vi "AuMT8852B Initial Carrier Test Configuration.vi"(5 "Settings":T1={"Low frequency selection"=enum."Use low frequency", "Medium frequency selection"=enum."Use medium frequency", "High frequency selection"=enum."Use high frequency", "Low TX frequency"=2402.0, "Medium TX frequency"=2441.0, "High TX frequency"=2480.0, "Number of packets"=10, "Hop selection"=enum."Test with hopping on", "Hop mode"=enum."Defined", "Test control"=enum."Loopback", "Maximum positive limit"=75000.0, "Maximum negative limit"=75000.0, "Low RX frequency"=2480.0, "Medium RX frequency"=2402.0, "High RX frequency"=2402.0}, 7 "Set/Get (Set)":enum16{"Set", "Get"}(ring), 8 "error in (no error)":errorcluster, 10 "Script (3)":i32=3, 11 "VISA session":refnum<visa-resource-name>) -> (0 "error out":errorcluster, 2 "error code":i32, 3 "VISA session out":refnum<visa-resource-name>, 4 "Settings out":T1={"Low frequency selection"=enum."Use low frequency", "Medium frequency selection"=enum."Use medium frequency", "High frequency selection"=enum."Use high frequency", "Low TX frequency"=0.0, "Medium TX frequency"=0.0, "High TX frequency"=0.0, "Number of packets"=0, "Hop selection"=enum."Test with hopping on", "Hop mode"=enum."Any", "Test control"=enum."Loopback", "Maximum positive limit"=0.0, "Maximum negative limit"=0.0, "Low RX frequency"=0.0, "Medium RX frequency"=0.0, "High RX frequency"=0.0})   [LabVIEW 2017]
doc: "Anritsu MT8852B Bluetooth Tester\n\nConfigures the instrument for the Initial Carrier test.\n\nINPUTS\nSet/Get - whether the values are being sent to or retrieved from the instrument.\nScript - which of the stored scripts (1-10) will be queried or configured. Scripts 1 and 2 are read-only.\nSettings - parameters of the test to be written.\n\nOUTPUTS\nSettings out - current parameters of the test."
uses:
  <instrlib>/aumt8852B/General/Utilities/MT8850 Test Parameters.ctl
  <instrlib>/aumt8852B/General/Utilities/MT8850 Frequency Units.ctl
panel:
  in  "Case Constant\n(See Context Help)":bool
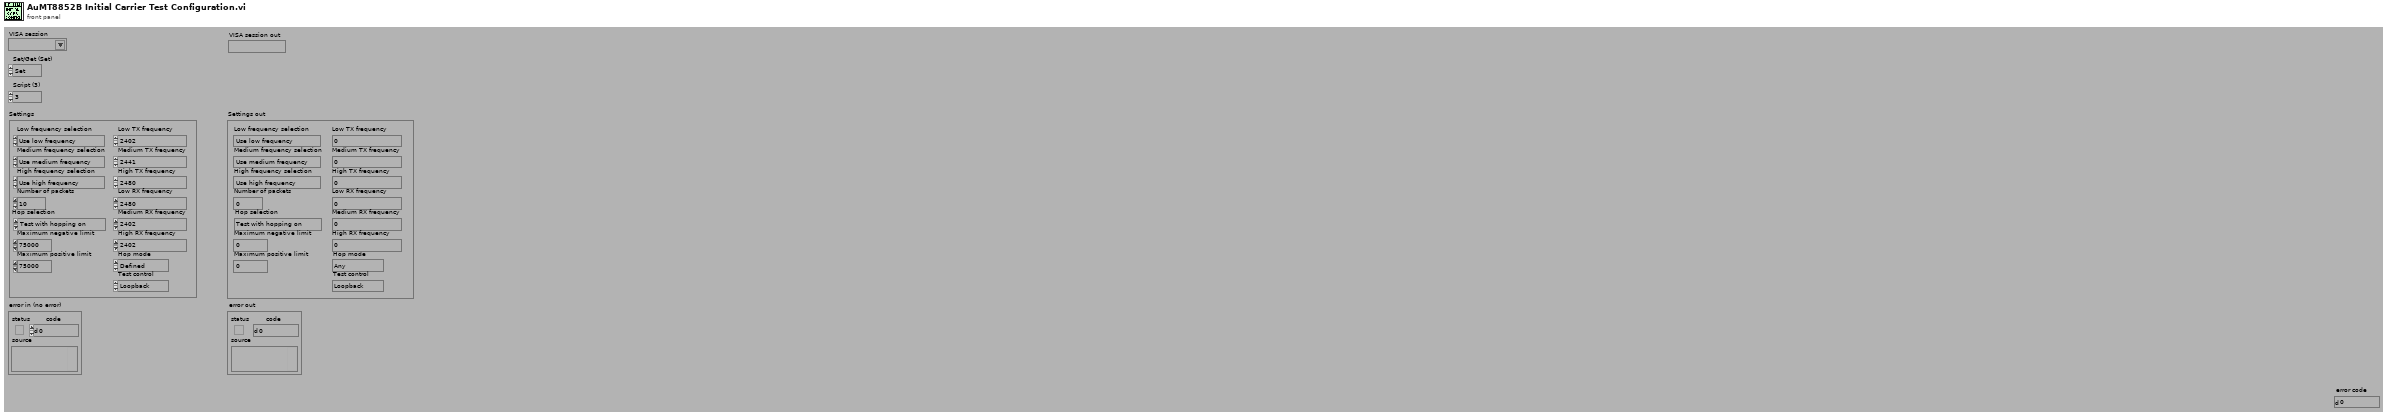
[diagram p1: front panel]
types:
  T1 = cluster{"Low frequency selection":enum16{"Don't use low frequency", "Use low frequency"}, "Medium frequency selection":enum16{"Don't use medium frequency", "Use medium frequency"}, "High frequency selection":enum16{"Don't use high frequency", "Use high frequency"}, "Low TX frequency":dbl, "Medium TX frequency":dbl, "High TX frequency":dbl, "Number of packets":i32, "Hop selection":enum16{"Test with hopping on", "Test with hopping off", "Test with hopping on and off"}, "Hop mode":enum16{"All", "Any", "Defined"}, "Test control":enum16{"Loopback", "TX test"}, "Maximum positive limit":dbl, "Maximum negative limit":dbl, "Low RX frequency":dbl, "Medium RX frequency":dbl, "High RX frequency":dbl}
  T2 = typedef "MT8850 Test Parameters.ctl" = enum16{"Use low frequency", "Use medium frequency", "Use high frequency", "Low TX frequency", "Low RX frquency", "Medium TX frequency", "Medium RX frequency", "High TX frequency", "High RX frequency", "Number of packets", "Average high limit", "Average low limit", "Peak power limit", "Max power step limit", "Min power step limit", "f1 average minimum", "f1 average maximum", "f2 maximum", "f1/f2 average maximum", "Hop selection", "Use DH1 packets", "Use DH3 packets", "Use DH5 packets", "1 slot packet drift limit", "3 slot packet drift limit", "5 slot packet drift limit", "Drift rate limit", "TX power level", "Frequency offset", "Symbol timing", "Modulation index", "BER limit", "FER limit", "Use averaging high limit", "Use averaging low limit", "Use peak power limit", "Packet type", "Test control", "Use max power step limit", "Use min power step limit", "Number of cycles", "Use f1 average maximum", "Use f1 average minimum", "Use f2 maximum", "Use f1/f2 average maximum", "Hop mode", "Maximum negative limit", "Maximum positive limit", "Use maximum negative limit", "Use maximum positive limit", "Use 1 slot packet drift limit", "Use 3 slot packet drift limit", "Use 5 slot packet drift limit", "Use drift rate limit", "Use BER limit", "Use FER limit", "Use dirty parameter table", "Use null packet drift limit", "Null packet drift limit", "Minimum power", "Power delay", "Packet count", "Payload toggle", "Output power level", "2DHX packet type", "3DHX packet type", "Number of blocks", "TX and RX low frequency", "TX and RX medium frequency", "TX and RX high frequency", "TX frequency", "RX frequency", "Threshold bit count", "Total test bit count", "Number of bits", "PDPSK to PGFSK lower limit", "PDPSK to PGFSK upper limit", "Initial frequency error upper limit", "Initial frequency error lower limit", "Frequency error upper limit", "Frequency error lower limit", "Block frequency error upper limit", "Block frequency error lower limit", "2Mbs RMS DEVM limit", "3Mbs RMS DEVM limit", "2Mbs Peak DEVM limit", "3Mbs Peak DEVM limit", "2Mbs 99% packets DEVM limit", "3Mbs 99% packets DEVM limit", "Percentage of no error packets limit", "Threshold error limit", "Total test error limit"}
  T3 = typedef "MT8850 Frequency Units.ctl" = enum16{"Channel", "Hz", "kHz", "MHz", "GHz"}
  T4 = enum16{"Simulate", "Range check", "Cache", "Query instrument status"}
  T5 = enum16{"Output power", "Power control", "Modulation characteristics", "Initial carrier", "Carrier drift", "Single slot sensitivity", "Multiple slot sensitivity", "Maximum input power"}
  T6 = enum16{"Test with hopping on", "Test with hopping off", "Test with hopping on and off"}
  T7 = enum16{"Don't use high frequency", "Use high frequency"}
  T8 = enum16{"Don't use medium frequency", "Use medium frequency"}
  T9 = enum16{"Don't use low frequency", "Use low frequency"}
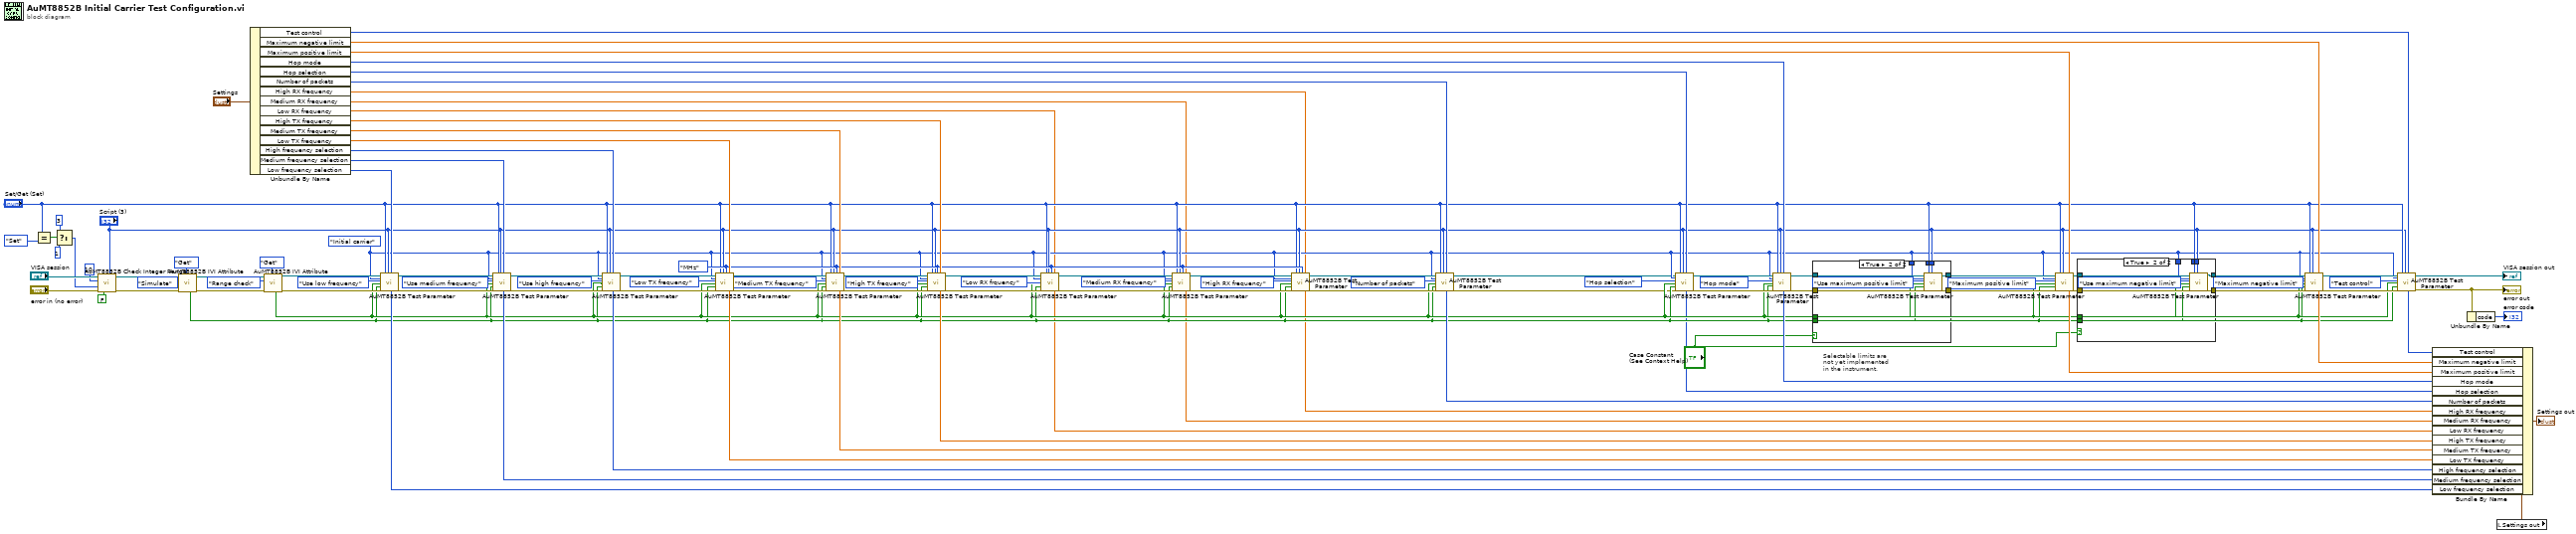
[diagram p0: block diagram]
diagram:
  w15 = MT8850_Frequency_Units."MHz" ("Frequency units (MHz)")
  w10 = T5."Initial carrier" ("Test (Output Power)")
  # "Selectable limits are\nnot yet implemented\nin the instrument."
  n1 = Equal?(x="Set/Get (Set)", y=enum16{"Set", "Get"}."Set") -> (x = y?=w106:bool)
  n2 = Select(t=3, s=w106, f=1) -> (s? t:f=w102:i32)
  n3 = call <instrlib>:"AuMT8852B Check Integer Range.vi"("Value (0)"="Script (3)", "Check IVI flag first? (T)"=FALSE, "error in (no error)"="error in (no error)", "Lower limit (-1)"=w102, "Upper limit (1)"=10, "VISA session"="VISA session") -> ("error out"=w100:errorcluster, "VISA session out"=w101:refnum<visa-resource-name>)  [unwired: 4 in]
  n4 = call <instrlib>:"AuMT8852B IVI Attribute.vi"("Set/Get (Set)"=enum16{"Set", "Get"}."Get", "error in (no error)"=w100, "Flag (Simulate)"=T4."Simulate", "VISA session"=w101) -> ("error out"=w81:errorcluster, "VISA session out"=w82:refnum<visa-resource-name>, "Value out"=w13:bool)  [unwired: 5 in]
  n5 = Unbundle By Name("Settings") -> ("Test control"=w43:enum16{"Loopback", "TX test"}, "Maximum negative limit"=w42:dbl, "Maximum positive limit"=w41:dbl, "Hop mode"=w60:enum16{"All", "Any", "Defined"}, "Hop selection"=w59:T6, "Number of packets"=w69:i32, "High RX frequency"=w9:dbl, "Medium RX frequency"=w8:dbl, "Low RX frequency"=w7:dbl, "High TX frequency"=w70:dbl, "Medium TX frequency"=w71:dbl, "Low TX frequency"=w72:dbl, "High frequency selection"=w73:T7, "Medium frequency selection"=w74:T8, "Low frequency selection"=w75:T9)
  n6 = call <instrlib>:"AuMT8852B IVI Attribute.vi"("Set/Get (Set)"=enum16{"Set", "Get"}."Get", "error in (no error)"=w81, "Flag (Simulate)"=T4."Range check", "VISA session"=w82) -> ("error out"=w79:errorcluster, "VISA session out"=w80:refnum<visa-resource-name>, "Value out"=w14:bool)  [unwired: 5 in]
  n7 = call <instrlib>:"AuMT8852B Test Parameter.vi"("VISA session"=w80, "Test (Output power)"=w10, "Parameter (Use low frequency)"=MT8850_Test_Parameters."Use low frequency", "Range check? (F)"=w14, "Simulate? (F)"=w13, "error in (no error)"=w79, "Set/Get (Set)"="Set/Get (Set)", "Script (3)"="Script (3)", "Integer value (0)"=w75) -> ("Integer value out"=w61:i32, "VISA session out"=w37:refnum<visa-resource-name>, "error out"=w36:errorcluster)  [unwired: 7 in, 1 out]
  n8 = call <instrlib>:"AuMT8852B Test Parameter.vi"("VISA session"=w37, "Test (Output power)"=w10, "Parameter (Use low frequency)"=MT8850_Test_Parameters."Use medium frequency", "Range check? (F)"=w14, "Simulate? (F)"=w13, "error in (no error)"=w36, "Set/Get (Set)"="Set/Get (Set)", "Script (3)"="Script (3)", "Integer value (0)"=w74) -> ("Integer value out"=w62:i32, "VISA session out"=w35:refnum<visa-resource-name>, "error out"=w34:errorcluster)  [unwired: 7 in, 1 out]
  n9 = call <instrlib>:"AuMT8852B Test Parameter.vi"("VISA session"=w35, "Test (Output power)"=w10, "Parameter (Use low frequency)"=MT8850_Test_Parameters."Use high frequency", "Range check? (F)"=w14, "Simulate? (F)"=w13, "error in (no error)"=w34, "Set/Get (Set)"="Set/Get (Set)", "Script (3)"="Script (3)", "Integer value (0)"=w73) -> ("Integer value out"=w63:i32, "VISA session out"=w96:refnum<visa-resource-name>, "error out"=w95:errorcluster)  [unwired: 7 in, 1 out]
  n10 = call <instrlib>:"AuMT8852B Test Parameter.vi"("VISA session"=w96, "Test (Output power)"=w10, "Parameter (Use low frequency)"=MT8850_Test_Parameters."Low TX frequency", "Range check? (F)"=w14, "Simulate? (F)"=w13, "error in (no error)"=w95, "Set/Get (Set)"="Set/Get (Set)", "Script (3)"="Script (3)", "Integer value (0)"=w15, "Float value (0)"=w72) -> ("Float value out"=w64:dbl, "VISA session out"=w94:refnum<visa-resource-name>, "error out"=w93:errorcluster)  [unwired: 6 in, 1 out]
  n11 = call <instrlib>:"AuMT8852B Test Parameter.vi"("VISA session"=w94, "Test (Output power)"=w10, "Parameter (Use low frequency)"=MT8850_Test_Parameters."Medium TX frequency", "Range check? (F)"=w14, "Simulate? (F)"=w13, "error in (no error)"=w93, "Set/Get (Set)"="Set/Get (Set)", "Script (3)"="Script (3)", "Integer value (0)"=w15, "Float value (0)"=w71) -> ("Float value out"=w65:dbl, "VISA session out"=w92:refnum<visa-resource-name>, "error out"=w91:errorcluster)  [unwired: 6 in, 1 out]
  n12 = call <instrlib>:"AuMT8852B Test Parameter.vi"("VISA session"=w92, "Test (Output power)"=w10, "Parameter (Use low frequency)"=MT8850_Test_Parameters."High TX frequency", "Range check? (F)"=w14, "Simulate? (F)"=w13, "error in (no error)"=w91, "Set/Get (Set)"="Set/Get (Set)", "Script (3)"="Script (3)", "Integer value (0)"=w15, "Float value (0)"=w70) -> ("Float value out"=w66:dbl, "VISA session out"=w17:refnum<visa-resource-name>, "error out"=w16:errorcluster)  [unwired: 6 in, 1 out]
  n13 = call <instrlib>:"AuMT8852B Test Parameter.vi"("VISA session"=w17, "Test (Output power)"=w10, "Parameter (Use low frequency)"=MT8850_Test_Parameters."Low RX frquency", "Range check? (F)"=w14, "Simulate? (F)"=w13, "error in (no error)"=w16, "Set/Get (Set)"="Set/Get (Set)", "Script (3)"="Script (3)", "Integer value (0)"=w15, "Float value (0)"=w7) -> ("Float value out"=w4:dbl, "VISA session out"=w19:refnum<visa-resource-name>, "error out"=w18:errorcluster)  [unwired: 6 in, 1 out]
  n14 = call <instrlib>:"AuMT8852B Test Parameter.vi"("VISA session"=w19, "Test (Output power)"=w10, "Parameter (Use low frequency)"=MT8850_Test_Parameters."Medium RX frequency", "Range check? (F)"=w14, "Simulate? (F)"=w13, "error in (no error)"=w18, "Set/Get (Set)"="Set/Get (Set)", "Script (3)"="Script (3)", "Integer value (0)"=w15, "Float value (0)"=w8) -> ("Float value out"=w5:dbl, "VISA session out"=w21:refnum<visa-resource-name>, "error out"=w20:errorcluster)  [unwired: 6 in, 1 out]
  n15 = call <instrlib>:"AuMT8852B Test Parameter.vi"("VISA session"=w21, "Test (Output power)"=w10, "Parameter (Use low frequency)"=MT8850_Test_Parameters."High RX frequency", "Range check? (F)"=w14, "Simulate? (F)"=w13, "error in (no error)"=w20, "Set/Get (Set)"="Set/Get (Set)", "Script (3)"="Script (3)", "Integer value (0)"=w15, "Float value (0)"=w9) -> ("Float value out"=w6:dbl, "VISA session out"=w22:refnum<visa-resource-name>, "error out"=w23:errorcluster)  [unwired: 6 in, 1 out]
  n16 = call <instrlib>:"AuMT8852B Test Parameter.vi"("VISA session"=w22, "Test (Output power)"=w10, "Parameter (Use low frequency)"=MT8850_Test_Parameters."Number of packets", "Range check? (F)"=w14, "Simulate? (F)"=w13, "error in (no error)"=w23, "Set/Get (Set)"="Set/Get (Set)", "Script (3)"="Script (3)", "Integer value (0)"=w69) -> ("Integer value out"=w67:i32, "VISA session out"=w2:refnum<visa-resource-name>, "error out"=w1:errorcluster)  [unwired: 7 in, 1 out]
  n17 = call <instrlib>:"AuMT8852B Test Parameter.vi"("VISA session"=w2, "Test (Output power)"=w10, "Parameter (Use low frequency)"=MT8850_Test_Parameters."Hop selection", "Range check? (F)"=w14, "Simulate? (F)"=w13, "error in (no error)"=w1, "Set/Get (Set)"="Set/Get (Set)", "Script (3)"="Script (3)", "Integer value (0)"=w59) -> ("Integer value out"=w3:i32, "VISA session out"=w90:refnum<visa-resource-name>, "error out"=w89:errorcluster)  [unwired: 7 in, 1 out]
  n18 = call <instrlib>:"AuMT8852B Test Parameter.vi"("VISA session"=w90, "Test (Output power)"=w10, "Parameter (Use low frequency)"=MT8850_Test_Parameters."Hop mode", "Range check? (F)"=w14, "Simulate? (F)"=w13, "error in (no error)"=w89, "Set/Get (Set)"="Set/Get (Set)", "Script (3)"="Script (3)", "Integer value (0)"=w60) -> ("Integer value out"=w58:i32, "VISA session out"=w27:refnum<visa-resource-name>, "error out"=w28:errorcluster)  [unwired: 7 in, 1 out]
  n19 = case shown="True" "Case Constant\n(See Context Help)" {
    tunnel: [w110 w120] -> w48
    tunnel: [w111 w119] -> w47
    tunnel: w28 -> [w110 w118]
    tunnel: w27 -> [w111 w117]
    tunnel: w14 -> [_ w116]
    tunnel: w13 -> [_ w115]
    tunnel: w10 -> [_ w114]
    tunnel: "Set/Get (Set)" -> [_ w113]
    tunnel: "Script (3)" -> [_ w112]
    frame False {
    }
    frame True {
      n20 = call <instrlib>:"AuMT8852B Test Parameter.vi"("VISA session"=w117, "Test (Output power)"=w114, "Parameter (Use low frequency)"=MT8850_Test_Parameters."Use maximum positive limit", "Range check? (F)"=w116, "Simulate? (F)"=w115, "error in (no error)"=w118, "Set/Get (Set)"=w113, "Script (3)"=w112) -> ("VISA session out"=w119:refnum<visa-resource-name>, "error out"=w120:errorcluster)  [unwired: 8 in, 2 out]
    }
  }
  n21 = call <instrlib>:"AuMT8852B Test Parameter.vi"("VISA session"=w47, "Test (Output power)"=w10, "Parameter (Use low frequency)"=MT8850_Test_Parameters."Maximum positive limit", "Range check? (F)"=w14, "Simulate? (F)"=w13, "error in (no error)"=w48, "Set/Get (Set)"="Set/Get (Set)", "Script (3)"="Script (3)", "Float value (0)"=w41) -> ("Float value out"=w44:dbl, "VISA session out"=w52:refnum<visa-resource-name>, "error out"=w49:errorcluster)  [unwired: 7 in, 1 out]
  n22 = case shown="True" "Case Constant\n(See Context Help)" {
    tunnel: [w123 w132] -> w53
    tunnel: w52 -> [w123 w131]
    tunnel: [w122 w130] -> w50
    tunnel: w49 -> [w122 w129]
    tunnel: w14 -> [_ w128]
    tunnel: w13 -> [_ w127]
    tunnel: w10 -> [_ w126]
    tunnel: "Set/Get (Set)" -> [_ w125]
    tunnel: "Script (3)" -> [_ w124]
    frame False {
    }
    frame True {
      n23 = call <instrlib>:"AuMT8852B Test Parameter.vi"("VISA session"=w131, "Test (Output power)"=w126, "Parameter (Use low frequency)"=MT8850_Test_Parameters."Use maximum negative limit", "Range check? (F)"=w128, "Simulate? (F)"=w127, "error in (no error)"=w129, "Set/Get (Set)"=w125, "Script (3)"=w124) -> ("VISA session out"=w132:refnum<visa-resource-name>, "error out"=w130:errorcluster)  [unwired: 8 in, 2 out]
    }
  }
  n24 = call <instrlib>:"AuMT8852B Test Parameter.vi"("VISA session"=w53, "Test (Output power)"=w10, "Parameter (Use low frequency)"=MT8850_Test_Parameters."Maximum negative limit", "Range check? (F)"=w14, "Simulate? (F)"=w13, "error in (no error)"=w50, "Set/Get (Set)"="Set/Get (Set)", "Script (3)"="Script (3)", "Float value (0)"=w42) -> ("Float value out"=w45:dbl, "VISA session out"=w54:refnum<visa-resource-name>, "error out"=w51:errorcluster)  [unwired: 7 in, 1 out]
  n25 = call <instrlib>:"AuMT8852B Test Parameter.vi"("VISA session"=w54, "Test (Output power)"=w10, "Parameter (Use low frequency)"=MT8850_Test_Parameters."Test control", "Range check? (F)"=w14, "Simulate? (F)"=w13, "error in (no error)"=w51, "Set/Get (Set)"="Set/Get (Set)", "Script (3)"="Script (3)", "Integer value (0)"=w43) -> ("Integer value out"=w46:i32, "VISA session out"=→"VISA session out":refnum<visa-resource-name>, "error out"=w30:errorcluster)  [unwired: 7 in, 1 out]
  "error out" <- w30
  n26 = Unbundle By Name(w30) -> ("code"=→"error code":i32)
  n27 = local read "Settings out"() -> (w68:T1)
  n28 = Bundle By Name(cluster=w68, "Test control"=w46, "Maximum negative limit"=w45, "Maximum positive limit"=w44, "Hop mode"=w58, "Hop selection"=w3, "Number of packets"=w67, "High RX frequency"=w6, "Medium RX frequency"=w5, "Low RX frequency"=w4, "High TX frequency"=w66, "Medium TX frequency"=w65, "Low TX frequency"=w64, "High frequency selection"=w63, "Medium frequency selection"=w62, "Low frequency selection"=w61) -> (→"Settings out":T1)
